vi "SetPersistentConfiguration.vi"(8 "ErrorIn":errorcluster, 9 "DataIn":variant, 11 "ReferenceIn":refnum<class "TraceWindow.lvclass">) -> (0 "ErrorOut":errorcluster, 1 "DataOut":variant, 3 "ReferenceOut":refnum<class "TraceWindow.lvclass">)   [LabVIEW 2021, in "TraceWindow.lvlib" / "TraceWindow.lvclass"]
uses:
  TraceWindow.lvclass
  a2d9dd7e-4f73-47a2-b010-087cab1955c7.vi
  f84ae1b1-18a6-43f0-8a99-6426ff7357f9.vi
  <vilib>/Utility/LVClass/Get LV Class Name.vi
  protected/MainGUIRepository.vi
  Library_TAF_ApplicationFramework/TAFBaseGUI/TAFBaseGUI.lvclass
  TraceWindow.lvclass/TraceWindow.ctl
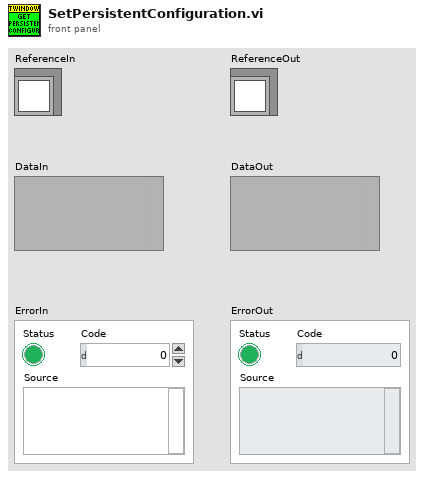
[diagram p1: front panel]
types:
  T1 = typedef "TraceWindow.lvlib/TraceWindow.lvclass/ObjectAttributes.ctl" = cluster{"Interfaces":cluster{"Dummys":refnum<class>}, "Locals":cluster{"MainGUIActive":refnum<queue>, "TraceQueue":refnum<queue>}, "Persistent":cluster{"OpenAtClosure":bool, "BufferSize":i32, "Startup":cluster{"OpenAtStartUp":bool, "OpenMinimized":bool}}}
  T2 = cluster{"OpenAtClosure":bool, "BufferSize":i32, "Startup":cluster{"OpenAtStartUp":bool, "OpenMinimized":bool}}
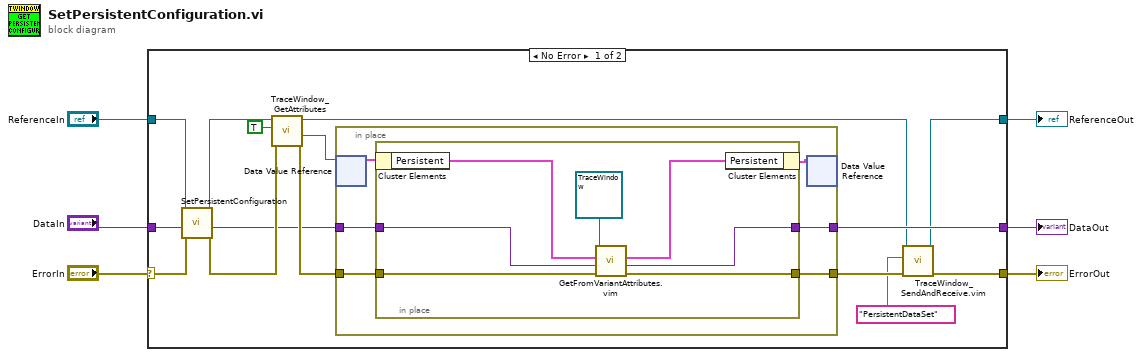
[diagram p0: block diagram]
diagram:
  n1 = case shown="No Error" "ErrorIn" {
    selector: "ErrorIn" -> [w19 w37]
    tunnel: [w17 w37] -> w5
    tunnel: [w8 w36] -> w3
    tunnel: "ReferenceIn" -> [w10 w36]
    tunnel: [w16 w35] -> w2
    tunnel: "DataIn" -> [w12 w35]
    frame No Error {
      n2 = call-parent "SetPersistentConfiguration.vi"("ErrorIn"=w19, "DataIn"=w12, "ReferenceIn"=w10) -> ("ErrorOut"=w18:errorcluster, "DataOut"=w13:variant, "ReferenceOut"=w11:refnum<class "TraceWindow.lvclass">)  [unwired: 6 in]
      n3 = call "TraceWindow_GetAttributes.vi"("ErrorIn"=w18, "OnlyGetDvrReference(False)"=TRUE, "ReferenceIn"=w11) -> ("ErrorOut"=w21:errorcluster, "DataRef"=w14:refnum<data-value>, "ReferenceOut"=w9:refnum<class "TraceWindow.lvclass">)  [unwired: 5 in, 1 out]
      n4 = in-place {
        in-place-border: w21 -> [w27]
        in-place-border: [w26] -> w20
        in-place-border: w13 -> [w25]
        in-place-border: [w24] -> w16
        n5 = in-place-dvr #1(w14) -> (w23:T1)  [unwired: 1 out]
        n6 = in-place {
          in-place-border: w27 -> [w34]
          in-place-border: [w33] -> w26
          in-place-border: w25 -> [w32]
          in-place-border: [w31] -> w24
          n7 = in-place-cluster #2(w23) -> ("Persistent"=w29:T2)
          n8 = call "GetFromVariantAttributes.vim"("ErrorIn"=w34, "DataInIn"=w32, "PersistentDataType"=w29, "Object"=refnum<class "TraceWindow.lvclass"> refnum ("VerticalButtonBar")) -> ("ErrorOut"=w33:errorcluster, "DataOut"=w31:variant, "PersistentDataOut"=w28:T2)  [unwired: 5 in]
          n9 = in-place-cluster #2("Persistent"=w28) -> (w22:T1)
        }
        n10 = in-place-dvr #1(w22) -> ()  [unwired: 2 out]
      }
      n11 = call "TraceWindow_SendAndReceive.vim"("ErrorIn"=w20, "Command"="PersistentDataSet", "ReferenceIn"=w9) -> ("ErrorOut"=w17:errorcluster, "ReferenceOut"=w8:refnum<class "TraceWindow.lvclass">)  [unwired: 6 in, 1 out]
    }
    frame Error {
    }
  }
  "ErrorOut" <- w5
  "ReferenceOut" <- w3
  "DataOut" <- w2
